vi "PH_BL-Master.get Boolean Status Service Subscriber Status.vi"(0 "i ref in":refnum<vi>, 2 "Index of wanted element":i32, 5 "error in (no error)":errorcluster) -> (8 "Wanted Boolean Ref":refnum<vi>, 11 "no Link?":bool, 13 "Information found?":bool, 14 "i ref out":refnum<vi>, 15 "off/false/out?":bool, 16 "on/true/in?":bool, 17 "Subscriber State":T1 items=["no info", "off/false/out", "on/true/in", "Failure", "Alarm", "Status 1", "Status 2", "Status 3"], 18 "off/false/out or on/true/in?":bool, 19 "error out":errorcluster)   [LabVIEW 2014, in "PH_BL-Master.lvlib"]
doc: "This VI gets the status of the selected Subscriber."
uses:
  PH_BL-Master.lvlib
  PH_StatusHandler/PH_StatusHandler.Status.ctl
  PH_StatusHandler/PH_StatusHandler.lvlib
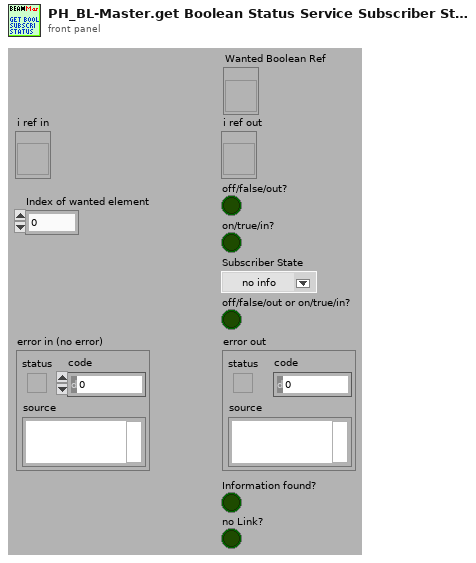
[diagram p1: front panel]
types:
  T1 = typedef "PH_StatusHandler.lvlib/PH_StatusHandler.Status.ctl" = i16
  T2 = typedef "PH_BL-Master.lvlib/PH_BL-Master.i attribute.ctl" = cluster{"Remote controlled":bool, "Boolean Condition Service Subscriber":refnum<vi>[], "Picture Condition Service Subscriber":refnum<vi>[], "R2S":cluster{"GUI Ref":refnum<vi>, "State":bool}, "Vacua":cluster{"GUI Ref":refnum<vi>, "Limit":dbl, "Curr Value":dbl, "in range":bool}[], "O2 Inspection":cluster{"GUI Ref":refnum<vi>, "Concentration":dbl, "State":T1}[], "Boolean Status Service Subscriber":cluster{"GUI Ref":refnum<vi>, "Status":T1, "no Link?":bool, "Status Subscriber Class":T3}[], "Picture Status Service Subscriber":cluster{"GUI Ref":refnum<vi>, "Status":T1, "no Link?":bool, "Status Subscriber Class":T3}[], "6P 4Q Service Subscriber":cluster{"GUI Ref":refnum<vi>, "Selector":T4, "no Link?":bool}[], "Index of latest 6P 4Q changing Instance":i32, "Index of latest Picture Status changing Instance":i32, "Index of latest Boolean Status changing Instance":i32, "Vision ID on same Node":string, "Start Phase over?":bool, "GUI Ref Delete":refnum<vi>}
  T3 = typedef "PH_BL-Master.lvlib/PH_BL-Master.Status Subscriber Class.ctl" = enum16{"unknown", "Switch", "BB", "6P Switch", "Switch GUI", "Switch and 6P State", "Force Sensor"}
  T4 = typedef "PH_4_Pos_Selector.lvlib/PH_4_Pos_Selector.Position Selector.ctl" = u16
  T5 = cluster{"GUI Ref":refnum<vi>, "Status":T1, "no Link?":bool, "Status Subscriber Class":T3}[]
  T6 = cluster{"GUI Ref":refnum<vi>, "Status":T1, "no Link?":bool, "Status Subscriber Class":T3}
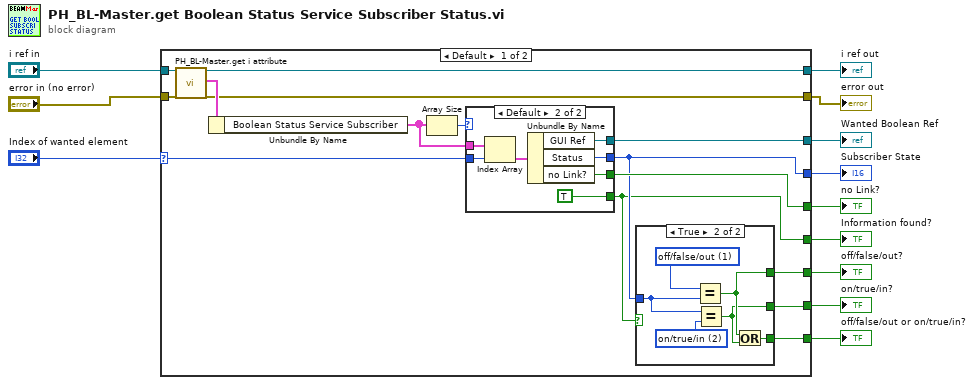
[diagram p0: block diagram]
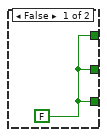
[diagram p2: hidden frame]
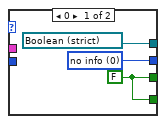
[diagram p3: hidden frame]
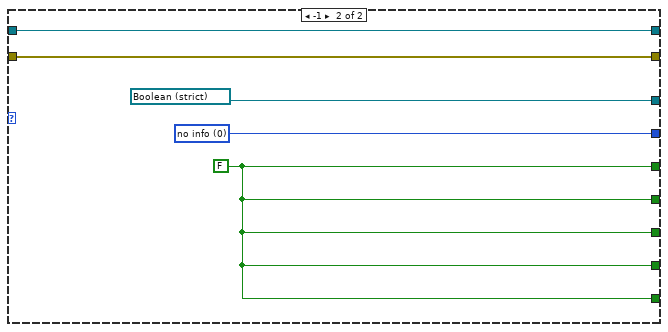
[diagram p4: hidden frame]
diagram:
  n1 = case shown="Default" "Index of wanted element" {
    selector: "Index of wanted element" -> [w15 _]
    tunnel: "error in (no error)" -> [w26 w48]
    tunnel: "i ref in" -> [w25 w49]
    tunnel: [w24 w49] -> w5
    tunnel: [w14 w47] -> w7
    tunnel: [w16 w48] -> w6
    tunnel: [w21 w45] -> w8
    tunnel: [w20 w45] -> w9
    tunnel: [w19 w45] -> w10
    tunnel: [w13 w45] -> w4
    tunnel: [w17 w45] -> w3
    tunnel: [w18 refnum<vi> refnum ("GUI Ref")] -> w2
    frame Default {
      n2 = call "PH_BL-Master.get i attribute.vi"("i ref in"=w25, "error in (no error)"=w26) -> ("i ref out"=w24:refnum<vi>, "i attribute"=w27:T2, "error out"=w16:errorcluster)  [unwired: 15 in]
      n3 = Unbundle By Name(w27) -> ("Boolean Status Service Subscriber"=w22:T5)
      n4 = Array Size(array=w22) -> (size(s)=w23:i32)
      n5 = case shown="Default" w23 {
        tunnel: w22 -> [_ w44]
        tunnel: [w37 w41] -> w14
        tunnel: [w35 TRUE] -> w13
        tunnel: [w35 w42] -> w17
        tunnel: [refnum<vi> refnum ("GUI Ref") w39] -> w18
        tunnel: w15 -> [_ w40]
        frame 0 {
          w35 = FALSE
          w37 = T1 0 items=["no info", "off/false/out", "on/true/in", "Failure", "Alarm", "Status 1", "Status 2", "Status 3"] ("State")
        }
        frame Default {
          n6 = Index Array(array=w44, index=w40) -> (element=w43:T6)
          n7 = Unbundle By Name(w43) -> ("GUI Ref"=w39:refnum<vi>, "Status"=w41:T1, "no Link?"=w42:bool)
        }
      }
      n8 = case shown="True" w13 {
        tunnel: [w28 w33] -> w21
        tunnel: [w28 w32] -> w20
        tunnel: [w28 w31] -> w19
        tunnel: w14 -> [_ w29]
        frame False {
          w28 = FALSE
        }
        frame True {
          w34 = T1 2 items=["no info", "off/false/out", "on/true/in", "Failure", "Alarm", "Status 1", "Status 2", "Status 3"] ("y")
          w30 = T1 1 items=["no info", "off/false/out", "on/true/in", "Failure", "Alarm", "Status 1", "Status 2", "Status 3"] ("y")
          n9 = Equal?(x=w30, y=w29) -> (x = y?=w33:bool)
          n10 = Equal?(x=w29, y=w34) -> (x = y?=w32:bool)
          n11 = Or(x=w33, y=w32) -> (x .or. y?=w31:bool)
        }
      }
    }
    frame -1 {
      w45 = FALSE
      w47 = T1 0 items=["no info", "off/false/out", "on/true/in", "Failure", "Alarm", "Status 1", "Status 2", "Status 3"] ("State")
    }
  }
  "i ref out" <- w5
  "error out" <- w6
  "Subscriber State" <- w7
  "off/false/out?" <- w8
  "on/true/in?" <- w9
  "off/false/out or on/true/in?" <- w10
  "Information found?" <- w4
  "no Link?" <- w3
  "Wanted Boolean Ref" <- w2
